vi "Server_Progetto.vi"() -> ()   [LabVIEW 2023]
uses:
  <vilib>/DAQmx/read.llb/DAQmx Read (Analog Wfm 1Chan NSamp).vi
  <vilib>/DAQmx/create/channels.llb/DAQmx Create Channel (AI-Voltage-Basic).vi
  <vilib>/DAQmx/configure/timing.llb/DAQmx Timing (Sample Clock).vi
  <vilib>/DAQmx/miscellaneous.llb/DAQmx Fill In Error Info.vi
panel:
  out "Messaggio letto":string
  out "Stato lettura":bool[](array[boolean])
  out "Stato scrittura":bool[](array[boolean])
  out "Lettura query":string
  out "Errore in uscita Letto":errorcluster
  out "Errore in uscita":errorcluster
  in  "byte di lettura":i32=50
  in  "Indirizzo":string="04"
  in  "Query":string="APPLY P25V,3.3,1.0; OUTP ON; APPL?; "
  in  "Errore ingresso":errorcluster
  out "Errore in uscita":errorcluster
  in  "Canale acquisizione":tag="Dev2/ai0"
  out "Tipo":dbl[](array[numeric]) format="%.2f"
  out "F.Campionamento":dbl format="%.2f"
  out "T.Osservazione":dbl format="%.2f"
  in  "Modalità di acquisizione":i32(ring)=10178 items=["Finite Samples"=10178, "Continuous Samples"=10123, "Hardware Timed Single Point"=12522]
  in  "VFs minimo":dbl=-5.0 format="%0.2f"
  in  "VFs massimo":dbl=5.0 format="%0.2f"
  out "Errore in uscita":errorcluster
  in  "Porta di comunicazione":u16=1000
  out "Indirizzo Client":string="localhost"
  # "COMUNICAZIONE"
  # "ACQUISIZIONE"
  # "ALIMENTAZIONE"
  # "PARAMETRI"
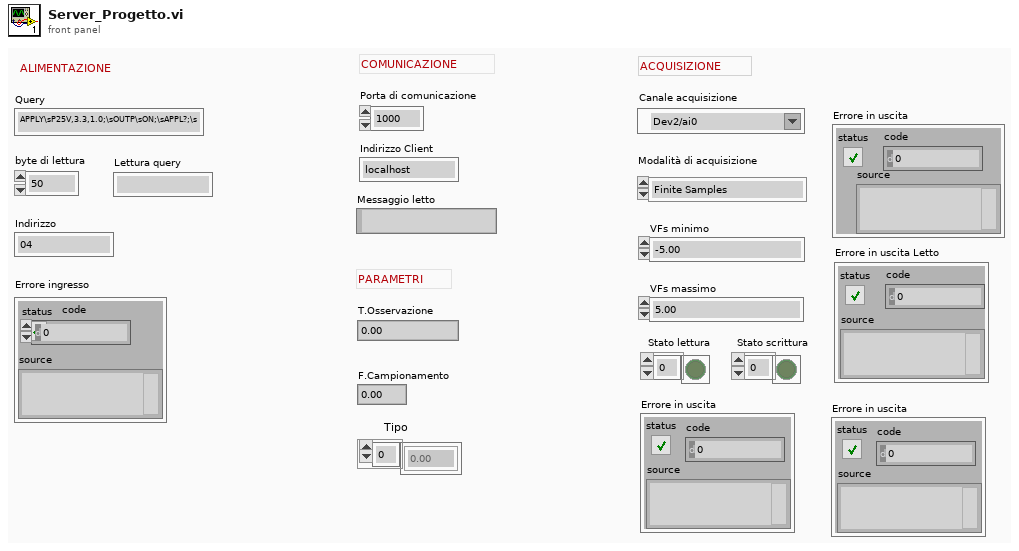
[diagram p1: front panel]
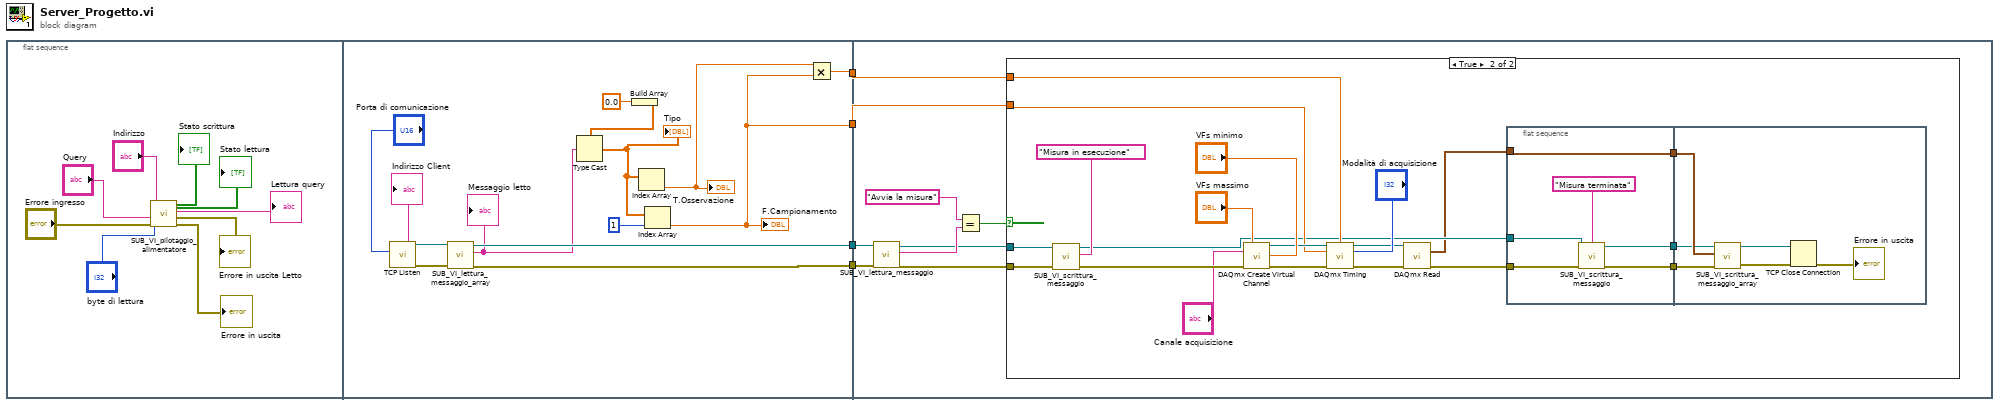
[diagram p0: block diagram]
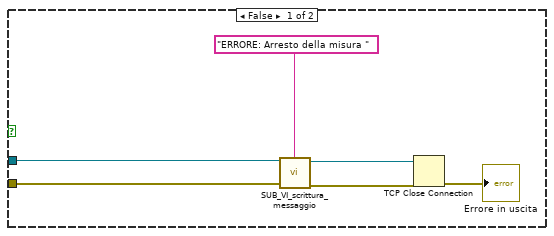
[diagram p2: hidden frame]
diagram:
  n1 = flat-sequence {
    tunnel: [w25] -> w4
    tunnel: [w16] -> w3
    tunnel: [w19] -> w2
    tunnel: [w15] -> w1
    tunnel: w4 -> [w31]
    tunnel: w3 -> [w30]
    tunnel: w2 -> [w29]
    tunnel: w1 -> [w28]
    frame #0 {
      n2 = call "SUB_VI_pilotaggio_alimentatore.vi"("Errore ingresso"="Errore ingresso", "Query"="Query", "Indirizzo"="Indirizzo", "byte di lettura"="byte di lettura") -> ("Errore in uscita"=→"Errore in uscita":errorcluster, "Errore in uscita Letto"=→"Errore in uscita Letto":errorcluster, "Lettura query"=→"Lettura query":string, "Stato scrittura"=→"Stato scrittura":bool[], "Stato lettura"=→"Stato lettura":bool[])  [unwired: 3 in]
    }
    frame #1 {
      n3 = call <vilib>:"TCP Listen.vi"("port"="Porta di comunicazione") -> ("error out"=w17:errorcluster, "remote address"=→"Indirizzo Client":string, "connection ID"=w18:refnum<k5>)  [unwired: 6 in, 2 out]
      n4 = call "SUB_VI_lettura_messaggio_array.vi"("Errore in ingresso"=w17, "TCP Network Connection in"=w18) -> ("Errore in uscita"=w16:errorcluster, "Messaggio letto"=w14:string, "TCP Network Connection out"=w15:refnum<k5>)  [unwired: 7 in]
      "Messaggio letto" <- w14
      n5 = Build Array(0.0) -> (w24:dbl[])
      n6 = Type Cast(type=w24, x=w14) -> (*(type *) &x=w21:dbl[])
      "Tipo" <- w21
      n7 = Index Array(array=w21) -> (element=w20:dbl)  [unwired: 1 in]
      "T.Osservazione" <- w20
      n8 = Index Array(array=w21, index=1) -> (element=w19:dbl)
      "F.Campionamento" <- w19
      n9 = Multiply(x=w20, y=w19) -> (x*y=w25:dbl)
    }
    frame #2 {
      n10 = call "SUB_VI_lettura_messaggio.vi"("Errore ingresso"=w30, "TCP Network Connection in"=w28) -> ("Errore uscita"=w33:errorcluster, "Messaggio ricevuto"=w36:string, "TCP Network Connection out"=w34:refnum<k5>)  [unwired: 6 in, 1 out]
      n11 = Equal?(x="Avvia la misura", y=w36) -> (x = y?=w32:bool)
      n12 = case shown="True" w32 {
        tunnel: w34 -> [w41 w62]
        tunnel: w33 -> [w40 w61]
        tunnel: w31 -> [_ w50]
        tunnel: w29 -> [_ w51]
        frame False {
          n13 = call "SUB_VI_scrittura_messaggio.vi"("Errore in ingresso"=w40, "Messaggio da inviare"="ERRORE: Arresto della misura " ("string"), "TCP Network \nConnection in"=w41) -> ("Errore in uscita"=w38:errorcluster, "TCP Network \nConnection out"=w39:refnum<k5>)  [unwired: 7 in]
          n14 = TCP Close Connection(connection ID=w39, error in (no error)=w38) -> (error out=→"Errore in uscita":errorcluster)  [unwired: 1 in, 1 out]
        }
        frame True {
          n15 = call "SUB_VI_scrittura_messaggio.vi"("Errore in ingresso"=w61, "Messaggio da inviare"="Misura in esecuzione" ("string"), "TCP Network \nConnection in"=w62) -> ("Errore in uscita"=w52:errorcluster, "TCP Network \nConnection out"=w47:refnum<k5>)  [unwired: 7 in]
          n16 = call-poly <vilib>:"DAQmx Create Virtual Channel.vi"("maximum value"="VFs massimo", "minimum value"="VFs minimo", "physical channels"="Canale acquisizione", "error in"=w52) -> ("task out"=w56:refnum<k21>, "error out"=w55:errorcluster)  [unwired: 10 in]
          n17 = call-poly <vilib>:"DAQmx Timing.vi"("task/channels in"=w56, "sample mode"="Modalità di acquisizione", "samples per channel"=w50, "rate"=w51, "error in"=w55) -> ("task out"=w53:refnum<k21>, "error out"=w54:errorcluster)  [unwired: 9 in]
          n18 = call-poly <vilib>:"DAQmx Read.vi"("task/channels in"=w53, "error in"=w54) -> ("data"=w45:waveform(dbl), "error out"=w48:errorcluster)  [unwired: 11 in, 1 out]
          n19 = flat-sequence {
            tunnel: w48 -> [w66]
            tunnel: w47 -> [w67]
            tunnel: [w68] -> w46
            tunnel: w45 -> [w68]
            tunnel: [w65] -> w44
            tunnel: [w64] -> w43
            tunnel: w46 -> [w71]
            tunnel: w44 -> [w70]
            tunnel: w43 -> [w69]
            frame #0 {
              n20 = call "SUB_VI_scrittura_messaggio.vi"("Errore in ingresso"=w66, "Messaggio da inviare"="Misura terminata" ("string"), "TCP Network \nConnection in"=w67) -> ("Errore in uscita"=w64:errorcluster, "TCP Network \nConnection out"=w65:refnum<k5>)  [unwired: 7 in]
            }
            frame #1 {
              n21 = call "SUB_VI_scrittura_messaggio_array.vi"("Errore in ingresso"=w69, "Segnale da inviare"=w71, "TCP Network Connection in"=w70) -> ("Errore uscita"=w72:errorcluster, "TCP Network Connection out"=w73:refnum<k5>)  [unwired: 7 in]
              n22 = TCP Close Connection(connection ID=w73, error in (no error)=w72) -> (error out=→"Errore in uscita":errorcluster)  [unwired: 1 in, 1 out]
            }
          }
        }
      }
    }
  }
